vi "Module Loop.vi"(8 "error in (no error)":errorcluster, 11 "Event Reporter Module in":refnum<class "Event Reporter Module.lvclass">) -> (0 "error out":errorcluster, 3 "Event Reporter Module out":refnum<class "Event Reporter Module.lvclass">)   [LabVIEW 2020, in "Volatus.lvlib" / "Event Reporter Module.lvclass"]
uses:
  Event Reporter Module.lvclass
  C:/dev/lv20CE/relink/lv-volatus/Volatus/Module/Module.lvclass
  Module/Module.lvclass/Module.ctl
  Event Reporter Module.lvclass/Event Reporter Module.ctl
  Module/Module.lvclass
  messages/Events/Class/Msg.lvclass
  C:/dev/lv20CE/relink/lv-protoc/LV-Proto/Message/Message.lvclass
  messages/Events/Class/Msg.lvclass/Msg.ctl
  VolatusAPI/VolatusAPI.lvclass/VolatusAPI.ctl
  VolatusConfig/VolatusConfigElement/VolatusConfigElement.lvclass/VolatusConfigElement.ctl
  Remote Messaging Identity/Remote Messaging Identity.lvclass
  C:/dev/lv20CE/relink/lv-volatus/Volatus/Identity/Identity.lvclass
  Event.ctl
  Event Level.ctl
  MessageQ/MessageQ.lvclass/MessageQ.ctl
  Events Summary.ctl
  MessageQ/MessageQ.lvclass
  PathValue/PathValue.lvclass/PathValue.ctl
  VolatusConfig/VolatusConfigElement/Element.vi
  VolatusConfig/Node/Node Config.lvclass
  C:/dev/lv20CE/relink/lv-volatus/VolatusConfig/VolatusConfigElement/VolatusConfigElement.lvclass
  <vilib>/Utility/error.llb/Error Cluster From Error Code.vi
  lv-promises/Promises/Promise/Promise.lvclass
  PathValue/PathValue.lvclass
  Volatus.lvlib
  VolatusAPI/VolatusAPI.lvclass
  Events Summary Value/Events Summary Value.lvclass
  VolatusConfig/Cluster/Cluster Config.lvclass
  VolatusConfig/VolatusConfigElement/VolatusConfigElement.lvclass
  C:/dev/lv20CE/relink/lv-volatus/Volatus/Event Reporter Module/Event Reporter Module.lvclass
  lv-exec-anchor/ExecAnchor/ExecAnchor.lvclass
  C:/dev/lv20CE/relink/lv-volatus/messages/Events/Class/Msg.lvclass
  C:/dev/lv20CE/relink/lv-volatus/VolatusConfig/Node/Node Config.lvclass
  C:/dev/lv20CE/relink/lv-volatus/Volatus/Remote Messaging Identity/Remote Messaging Identity.lvclass
panel:
  # "Event Reporter"
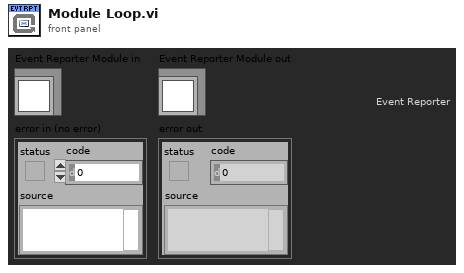
[diagram p1: front panel]
types:
  T1 = enum32{"Invalid", "Standard", "Closed", "Hidden", "Minimized", "Maximized"}
  T2 = typedef "Volatus.lvlib/Event.ctl" = cluster{"Time Stamp":timestamp, "Event Level":T3, "Context":string, "Message":string, "Error":errorcluster, "Node":string}
  T3 = typedef "Volatus.lvlib/Event Level.ctl" = enum16{"Debug", "Info", "Warning", "Error"}
  T4 = typedef "Volatus.lvlib/Events Summary.ctl" = cluster{"# Debug":i32, "# Info":i32, "# Warning":i32, "# Error":i32}
  T5 = typedef "TcpPayload.lvlib/Data.ctl" = cluster{"target_node":u32, "source_id":u32, "sequence":u32, "timestamp":i64, "type":string, "task_id":string, "payload":u8[]}
  T6 = typedef "Events.lvlib/Data.ctl" = cluster{"events":T7[]}
  T7 = typedef "Event.lvlib/Data.ctl" = cluster{"timestamp":i64, "level":T8, "context":string, "message":string, "error":T9}
  T8 = typedef "EventLevel.lvlib/Enumeration.ctl" = enum16{"EVENTLEVEL_UNKNOWN", "EVENTLEVEL_DEBUG", "EVENTLEVEL_INFO", "EVENTLEVEL_WARNING", "EVENTLEVEL_ERROR"}
  T9 = typedef "Error.lvlib/Data.ctl" = errorcluster
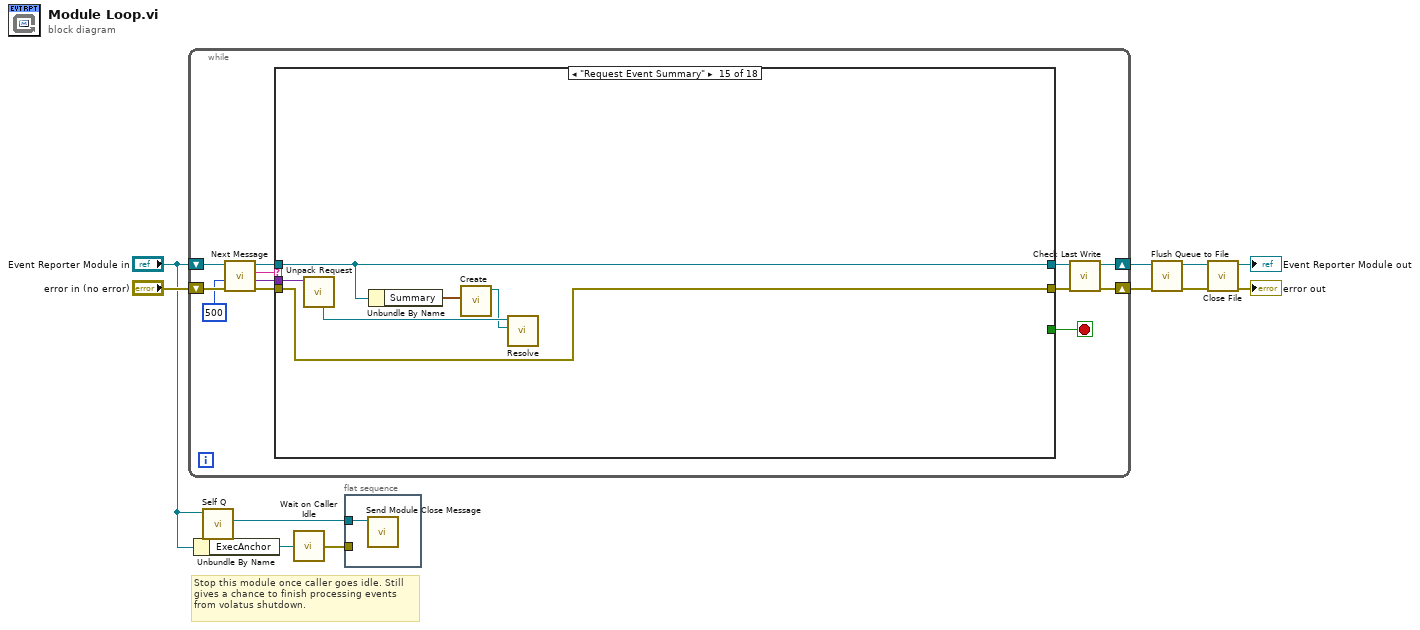
[diagram p0: block diagram]
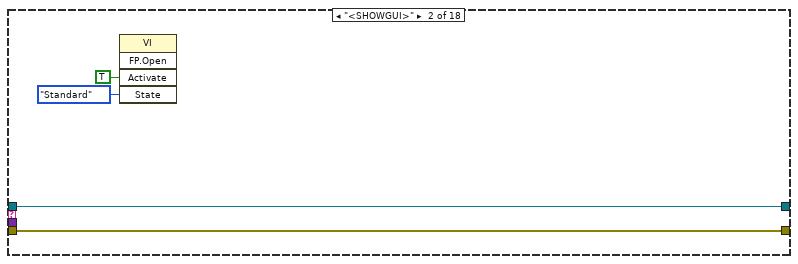
[diagram p3: hidden frame]
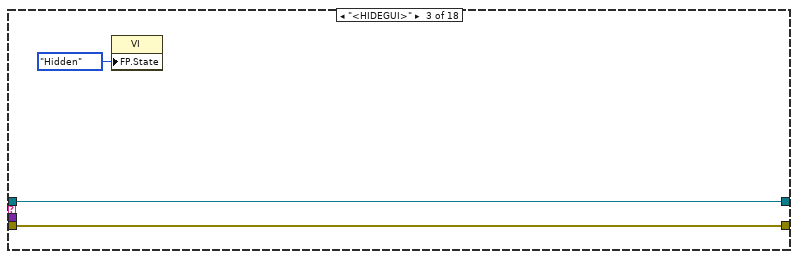
[diagram p4: hidden frame]
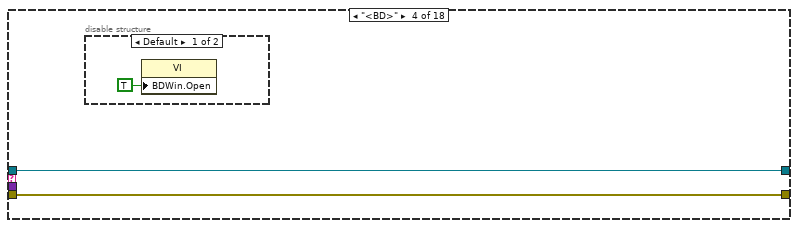
[diagram p5: hidden frame]
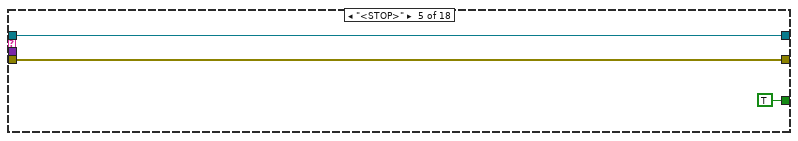
[diagram p7: hidden frame]
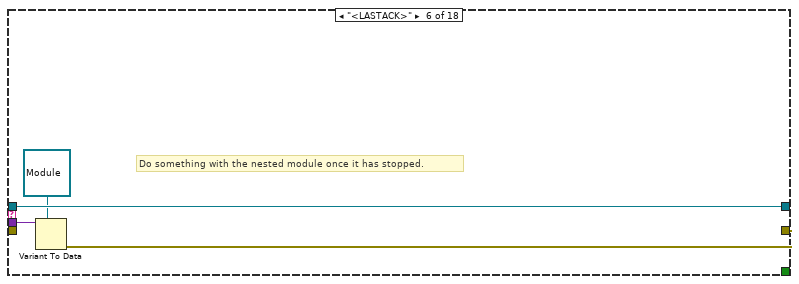
[diagram p8: hidden frame]
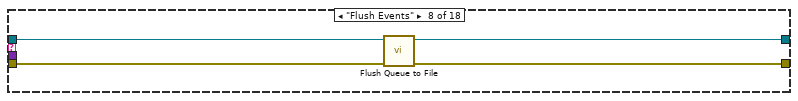
[diagram p10: hidden frame]
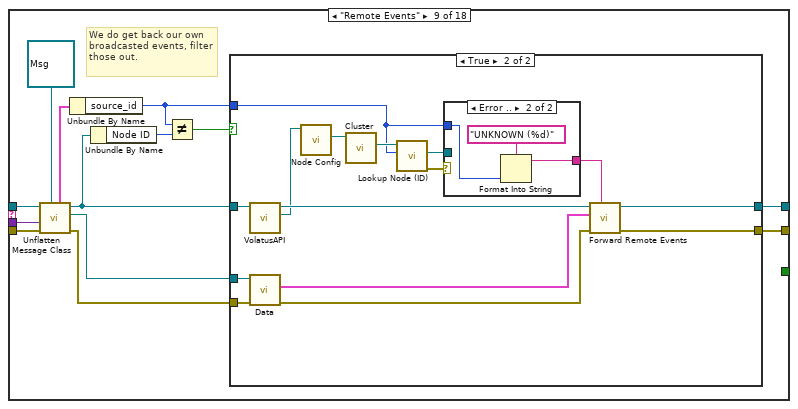
[diagram p11: hidden frame]
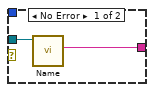
[diagram p13: hidden frame]
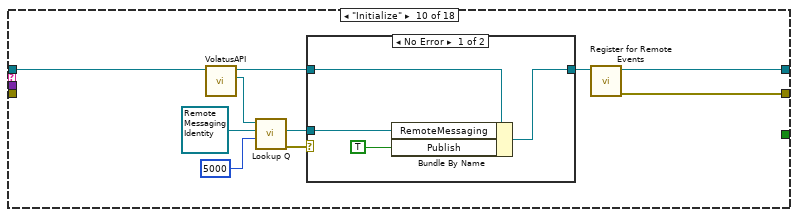
[diagram p14: hidden frame]
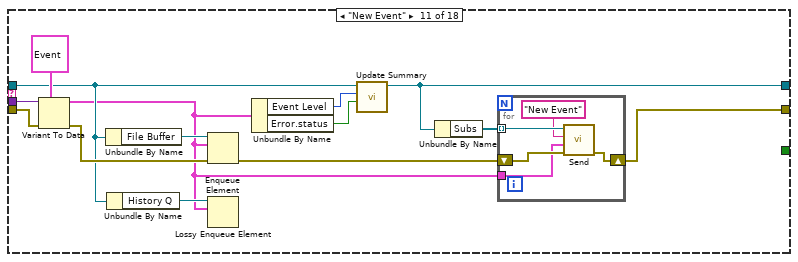
[diagram p16: hidden frame]
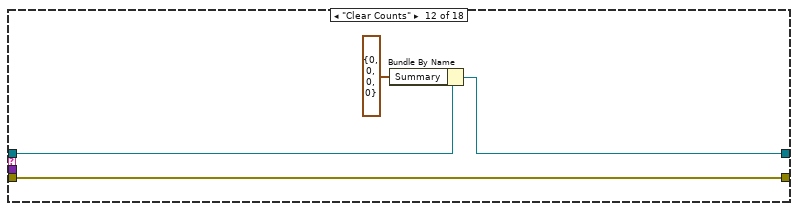
[diagram p17: hidden frame]
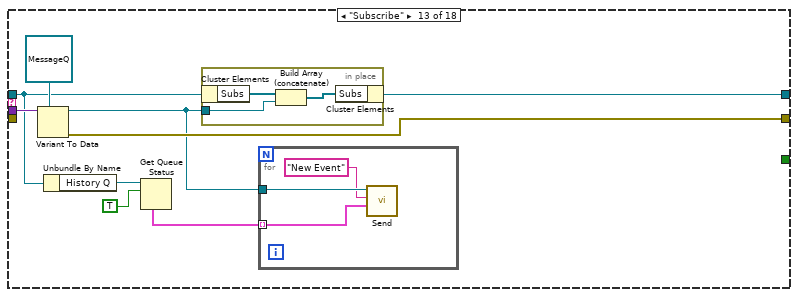
[diagram p18: hidden frame]
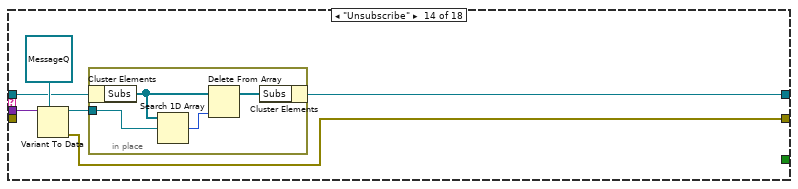
[diagram p19: hidden frame]
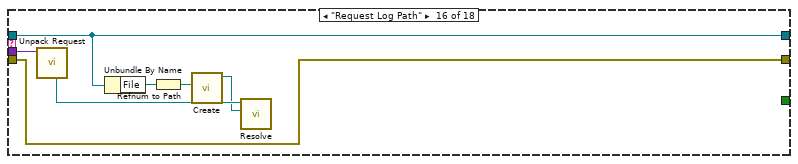
[diagram p20: hidden frame]
diagram:
  # "Stop this module once caller goes idle. Still gives a chance to finish processing events from volatus shutdown."
  n1 = while {
    shift-right: [w14] -> w8
    shift-left: "Event Reporter Module in" -> [w23]
    shift-right: [w16] -> w11
    shift-left: "error in (no error)" -> [w22]
    stop <- w18 stop-if-true
    n2 = call "Next Message.vi"("error in (no error)"=w22, "Timeout ms (-1)"=500, "Module in"=w23) -> ("error out"=w21:errorcluster, "Data"=w17:variant, "ID"=w20:string, "Module out"=w19:refnum<class "Event Reporter Module.lvclass">)  [unwired: 5 in]
    n3 = case shown="\"Request Event Summary\"" w20 {
      tunnel: w21 -> [w24 w26 w31 w33 w36 _ w44 w48 w61 _ w110 w119 _ _ w147 w153 w163 w167]
      tunnel: w19 -> [w25 w29 w32 w34 w38 w42 w43 w46 w60 w91 w107 w121 w126 w140 w149 w158 w161 w165]
      tunnel: [w25 w29 w32 w34 w38 w42 w43 w45 w54 w92 w105 w120 w127 w138 w149 w158 w160 w164] -> w15
      tunnel: [_ _ _ _ TRUE _ _ _ _ _ _ _ _ _ _ _ _ _] -> w18
      tunnel: w17 -> [_ _ _ _ _ w41 _ _ w59 _ w112 _ w130 w142 w152 w159 _ _]
      tunnel: [w24 w26 w31 w33 w36 w39 w44 w47 w53 w93 w102 w119 w128 w137 w147 w153 w162 w166] -> w13
      frame "<CLOSE>" {
        # "If the module might be in a state that can be stopped, add logic to decide whether or not to actually stop."
        # "Add additional code to handle stopping the module."
      }
      frame "<SHOWGUI>" {
        n4 = invoke class="VI" method="FP.Open"("Activate"=TRUE ("Activate?"), "State"=T1."Standard") -> ()  [unwired: 3 in, 5 out]
      }
      frame "<HIDEGUI>" {
        n5 = property class="VI"("FP.State"=T1."Hidden" ("Front Panel Window:State")) -> ()  [unwired: 2 in, 2 out]
      }
      frame "<BD>" {
        n6 = disable-structure shown="Default" {
          frame condition #0 (active) {
            n7 = property class="VI"("BDWin.Open"=TRUE ("Block Diagram Window:Open")) -> ()  [unwired: 2 in, 2 out]
          }
          frame condition #1 {
          }
        }
      }
      frame "<STOP>" {
      }
      frame "<LASTACK>" {
        # "Do something with the nested module once it has stopped."
        n8 = Variant To Data(type=refnum<class "Module.lvclass"> refnum ("Volatus:Module"), Variant=w41) -> (error out=w39:errorcluster)  [unwired: 1 in, 1 out]
      }
      frame "<TIMEOUT>" {
        # "Need to spin to allow the Check Last Write.vi to enqueue a flush message if no new events are incoming."
      }
      frame "Flush Events" {
        n9 = call "Flush Queue to File.vi"("error in (no error)"=w48, "Event Reporter Module in"=w46) -> ("error out"=w47:errorcluster, "Event Reporter Module out"=w45:refnum<class "Event Reporter Module.lvclass">)  [unwired: 8 in]
      }
      frame "Remote Events" {
        # "We do get back our own broadcasted events, filter those out."
        n10 = call "Unflatten Message Class.vi"("Message Type"=refnum<class "Msg.lvclass"> refnum ("Events.lvlib:Msg.lvclass"), "error in (no error)"=w61, "Data"=w59, "Module in"=w60) -> ("error out"=w55:errorcluster, "Message"=w57:refnum<class "Msg.lvclass">, "Module out"=w50:refnum<class "Event Reporter Module.lvclass">, "TcpPayload"=w56:T5)  [unwired: 4 in]
        n11 = Unbundle By Name(w56) -> ("source_id"=w52:u32)
        n12 = Unbundle By Name(w50) -> ("Node ID"=w49:u32)
        n13 = Not Equal?(x=w52, y=w49) -> (x != y?=w51:bool)
        n14 = case shown="True" w51 {
          tunnel: w57 -> [_ w78]
          tunnel: w55 -> [w62 w77]
          tunnel: [w63 w65] -> w54
          tunnel: [w62 w67] -> w53
          tunnel: w50 -> [w63 w76]
          tunnel: w52 -> [_ w69]
          frame False {
          }
          frame True {
            n15 = call "VolatusAPI.vi"("Module in"=w76) -> ("VolatusAPI"=w74:refnum<class "VolatusAPI.lvclass">, "Module out"=w75:refnum<class "Event Reporter Module.lvclass">)  [unwired: 9 in]
            n16 = call "Data.vi"("error in (no error)"=w77, "PB Msg Template in"=w78) -> ("error out"=w68:errorcluster, "Data"=w64:T6)  [unwired: 7 in, 1 out]
            n17 = call "Node Config.vi"("VolatusAPI in"=w74) -> ("Node Config"=w73:refnum<class "Node Config.lvclass">)  [unwired: 9 in, 1 out]
            n18 = call "Cluster.vi"("Node in"=w73) -> ("Cluster"=w72:refnum<class "Cluster Config.lvclass">)  [unwired: 8 in, 2 out]
            n19 = call "Lookup Node (ID).vi"("Node ID"=w69, "Cluster in"=w72) -> ("error out"=w71:errorcluster, "Node"=w70:refnum<class "Node Config.lvclass">)  [unwired: 7 in, 1 out]
            n20 = case shown="Error .." w71 {
              tunnel: w70 -> [w80 _]
              tunnel: [w79 w81] -> w66
              tunnel: w69 -> [_ w82]
              frame No Error {
                n21 = call "Name.vi"("VolatusConfigElement in"=w80) -> ("Name"=w79:string)  [unwired: 8 in, 2 out]
              }
              frame Error {
                n22 = Format Into String(format string="UNKNOWN (%d)" ("Name"), w82) -> (resulting string=w81:string)  [unwired: 2 in, 1 out]
              }
            }
            n23 = call "Forward Remote Events.vi"("Node"=w66, "error in (no error)"=w68, "Data"=w64, "Event Reporter Module in"=w75) -> ("error out"=w67:errorcluster, "Event Reporter Module out"=w65:refnum<class "Event Reporter Module.lvclass">)  [unwired: 6 in]
          }
        }
      }
      frame "Initialize" {
        n24 = call "VolatusAPI.vi"("Module in"=w91) -> ("VolatusAPI"=w84:refnum<class "VolatusAPI.lvclass">, "Module out"=w90:refnum<class "Event Reporter Module.lvclass">)  [unwired: 9 in]
        n25 = call "Lookup Q.vi"("Timeout ms (0)"=5000, "Identity"=refnum<class "Remote Messaging Identity.lvclass"> refnum ("Volatus:Remote Messaging Identity.lvclass"), "VolatusAPI in"=w84) -> ("error out"=w87:errorcluster, "MessageQ"=w86:refnum<class "MessageQ.lvclass">)  [unwired: 6 in, 1 out]
        n26 = case shown="No Error" w87 {
          tunnel: w86 -> [w96 _]
          tunnel: w90 -> [w97 w98]
          tunnel: [w95 w98] -> w85
          frame No Error {
            n27 = Bundle By Name(cluster=w97, "RemoteMessaging"=w96, "Publish"=TRUE) -> (w95:refnum<class "Event Reporter Module.lvclass">)
          }
          frame Error {
          }
        }
        n28 = call "Register for Remote Events.vi"("Event Reporter Module in"=w85) -> ("error out"=w93:errorcluster, "Event Reporter Module out"=w92:refnum<class "Event Reporter Module.lvclass">)  [unwired: 9 in]
      }
      frame "New Event" {
        n29 = Variant To Data(error in=w110, type=T2 {"Time Stamp"=timestamp(0 s since 1904-01-01), "Event Level"=enum."Info", "Context"="", "Message"="", "Error"={"status"=FALSE, "code"=0, "source"=""}, "Node"=""} ("Event"), Variant=w112) -> (data=w101:T2, error out=w108:errorcluster)
        n30 = Unbundle By Name(w107) -> ("File Buffer"=w109:refnum<queue>)
        n31 = Unbundle By Name(w107) -> ("History Q"=w106:refnum<queue>)
        n32 = Enqueue Element(queue=w109, element=w101, error in (no error)=w108) -> (error out=w103:errorcluster)  [unwired: 1 in, 2 out]
        n33 = Lossy Enqueue Element(queue=w106, element=w101) -> ()  [unwired: 1 in, 4 out]
        n34 = Unbundle By Name(w101) -> ("Event Level"=w100:T3, "Error.status"=w99:bool)
        n35 = call "Update Summary.vi"("Error Status"=w99, "Level"=w100, "Event Reporter Module in"=w107) -> ("Event Reporter Module out"=w105:refnum<class "Event Reporter Module.lvclass">)  [unwired: 7 in, 1 out]
        n36 = Unbundle By Name(w105) -> ("Subs"=w104:refnum<class "MessageQ.lvclass">[])
        n37 = for {
          tunnel: w104 -> [w117] mode=indexing
          tunnel: w101 -> [w113]
          shift-right: [w115] -> w102
          shift-left: w103 -> [w116]
          n38 = call "Send.vi"("error in (no error)"=w116, "Data"=w113, "ID"="New Event", "MessageQ in"=w117) -> ("error out"=w115:errorcluster)  [unwired: 6 in, 1 out]
        }
      }
      frame "Clear Counts" {
        n39 = Bundle By Name(cluster=w121, "Summary"=T4 {"# Debug"=0, "# Info"=0, "# Warning"=0, "# Error"=0}) -> (w120:refnum<class "Event Reporter Module.lvclass">)
      }
      frame "Subscribe" {
        n40 = Variant To Data(type=refnum<class "MessageQ.lvclass"> refnum ("Volatus:MessageQ"), Variant=w130) -> (data=w122:refnum<class "MessageQ.lvclass">, error out=w128:errorcluster)  [unwired: 1 in]
        n41 = Unbundle By Name(w126) -> ("History Q"=w125:refnum<queue>)
        n42 = Get Queue Status(queue=w125, return elements? (F)=TRUE) -> (elements=w123:T2[])  [unwired: 1 in, 7 out]
        n43 = in-place {
          in-place-border: w122 -> [w135]
          n44 = in-place-cluster #1(w126) -> ("Subs"=w136:refnum<class "MessageQ.lvclass">[])
          n45 = Build Array (concatenate)(w136, w135) -> (w134:refnum<class "MessageQ.lvclass">[])
          n46 = in-place-cluster #1("Subs"=w134) -> (w127:refnum<class "Event Reporter Module.lvclass">)
        }
        n47 = for {
          tunnel: w123 -> [w131] mode=indexing
          tunnel: w122 -> [w133]
          n48 = call "Send.vi"("Data"=w131, "ID"="New Event", "MessageQ in"=w133) -> ()  [unwired: 7 in, 2 out]
        }
      }
      frame "Unsubscribe" {
        n49 = Variant To Data(type=refnum<class "MessageQ.lvclass"> refnum ("Volatus:MessageQ"), Variant=w142) -> (data=w139:refnum<class "MessageQ.lvclass">, error out=w137:errorcluster)  [unwired: 1 in]
        n50 = in-place {
          in-place-border: w139 -> [w146]
          n51 = in-place-cluster #2(w140) -> ("Subs"=w145:refnum<class "MessageQ.lvclass">[])
          n52 = Search 1D Array(1D array=w145, element=w146) -> (index of element=w144:i32)  [unwired: 1 in]
          n53 = Delete From Array(array=w145, index=w144) -> (array with subset deleted=w143:refnum<class "MessageQ.lvclass">[])  [unwired: 1 in, 1 out]
          n54 = in-place-cluster #2("Subs"=w143) -> (w138:refnum<class "Event Reporter Module.lvclass">)
        }
      }
      frame "Request Event Summary" {
        n55 = call "Unpack Request.vi"("Request Data"=w152) -> ("Promise"=w151:refnum<class "Promise.lvclass">)  [unwired: 8 in, 2 out]
        n56 = Unbundle By Name(w149) -> ("Summary"=w148:T4)
        n57 = call "Create.vi"("Events Summary"=w148) -> ("Events Summary Value out"=w150:refnum<class "Events Summary Value.lvclass">)  [unwired: 10 in]
        n58 = call "Resolve.vi"("Result (None)"=w150, "Promise in"=w151) -> ()  [unwired: 8 in, 2 out]
      }
      frame "Request Log Path" {
        n59 = call "Unpack Request.vi"("Request Data"=w159) -> ("Promise"=w155:refnum<class "Promise.lvclass">)  [unwired: 8 in, 2 out]
        n60 = Unbundle By Name(w158) -> ("File"=w157:refnum<file>)
        n61 = Refnum to Path(1:w157) -> (0:w156:path)
        n62 = call "Create.vi"("Path"=w156) -> ("PathValue out"=w154:refnum<class "PathValue.lvclass">)  [unwired: 10 in]
        n63 = call "Resolve.vi"("Result (None)"=w154, "Promise in"=w155) -> ()  [unwired: 8 in, 2 out]
      }
      frame "Split Log" {
        n64 = call "Split Log.vi"("error in (no error)"=w163, "Event Reporter Module in"=w161) -> ("error out"=w162:errorcluster, "Event Reporter Module out"=w160:refnum<class "Event Reporter Module.lvclass">)  [unwired: 8 in]
      }
      frame Default {
        n65 = call "Report Unhandled Message ID.vi"("error in (no error)"=w167, "Module in"=w165) -> ("error out"=w166:errorcluster, "Module out"=w164:refnum<class "Event Reporter Module.lvclass">)  [unwired: 8 in]
      }
    }
    n66 = call "Check Last Write.vi"("error in (no error)"=w13, "Event Reporter Module in"=w15) -> ("error out"=w16:errorcluster, "Event Reporter Module out"=w14:refnum<class "Event Reporter Module.lvclass">)  [unwired: 8 in]
  }
  n67 = Unbundle By Name("Event Reporter Module in") -> ("ExecAnchor"=w4:refnum<class "ExecAnchor.lvclass">)
  n68 = call "Self Q.vi"("Module in"="Event Reporter Module in") -> ("Self Q"=w1:refnum<class "MessageQ.lvclass">)  [unwired: 9 in, 1 out]
  n69 = call "Wait on Caller Idle.vi"("ExecAnchor in"=w4) -> ("error out"=w2:errorcluster)  [unwired: 4 in]
  n70 = flat-sequence {
    tunnel: w2 -> [_]
    tunnel: w1 -> [w168]
    frame #0 {
      n71 = call "Send Module Close Message.vi"("MessageQ"=w168) -> ()  [unwired: 10 in, 1 out]
    }
  }
  n72 = call "Flush Queue to File.vi"("error in (no error)"=w11, "Event Reporter Module in"=w8) -> ("error out"=w9:errorcluster, "Event Reporter Module out"=w6:refnum<class "Event Reporter Module.lvclass">)  [unwired: 8 in]
  n73 = call "Close File.vi"("error in (no error)"=w9, "Event Reporter Module in"=w6) -> ("error out"=→"error out":errorcluster, "Event Reporter Module out"=→"Event Reporter Module out":refnum<class "Event Reporter Module.lvclass">)  [unwired: 8 in]
